vi "IMAQ-MWT Contour SPINE TEST (FPGA).vi"() -> ()   [LabVIEW 2015]
uses:
  <vilib>/Platform/TimedLoop/XDataNode/wakeup.ctl
  <vilib>/Platform/TimedLoop/XDataNode/XDNodeRunTimeDep.lvlib
  <vilib>/Platform/TimedLoop/XDataNode/nitl_modes.ctl
  <vilib>/Platform/TimedLoop/XDataNode/timing_clust.ctl
  <vilib>/Platform/TimedLoop/XDataNode/XDataNode.xnode
  <vilib>/rvi/DataTransferAndStorage/Container/XNode/niFpgaContainer.xnode
  <vilib>/rvi/interface/RandomDataEmulation/nirviRandomDataFpgaReadWriteTemplate.vi
panel:
  in  "Clock Cycles Limit":u32=10000
  # "IMAQ - MWT"
  # "Edge, Contour and SPINE"
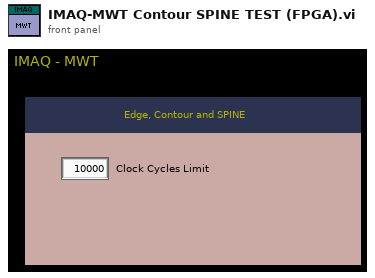
[diagram p1: front panel]
types:
  T1 = typedef "XDNodeRunTimeDep.lvlib/timing_clust.ctl" = cluster{"Expected End [f-1]":u64, "Actual End [f-1]":u64, "Finished Late? [f-1]":bool, "Expected End [i-1]":u64, "Actual End [i-1]":u64, "Finished Late? [i-1]":bool, "Expected Start [i]":u64, "Actual Start [i]":u64, "Expected Start [f]":u64, "Actual Start [f]":u64, "Source Name":string, "Structure Name":string, "Period":i64, "Deadline":i64, "Offset":i64, "Start":i64, "Priority":i32, "Timeout":i32, "Mode":T2, "Wakeup Reason":T3, "Error":errorcluster, "Source Type":string, "Secondary Source Type":string, "Global End Time":u64, "Global Start Time":u64, "Frame Duration":u64, "Iteration Duration":u64, "Assigned CPU":i32, "I/O Scan Engine Mode":u32}
  T2 = typedef "XDNodeRunTimeDep.lvlib/nitl_modes.ctl" = enum32{"No Change", "Process missed periods, maintain original phase", "Discard missed periods, maintain original phase", "Process missed periods, ignore original phase", "Discard missed periods, ignore original phase"}
  T3 = typedef "XDNodeRunTimeDep.lvlib/wakeup.ctl" = enum32{"Normal", "Aborted", "Asynchronous wakeup", "Timing source error", "Timed loop error", "Timeout"}
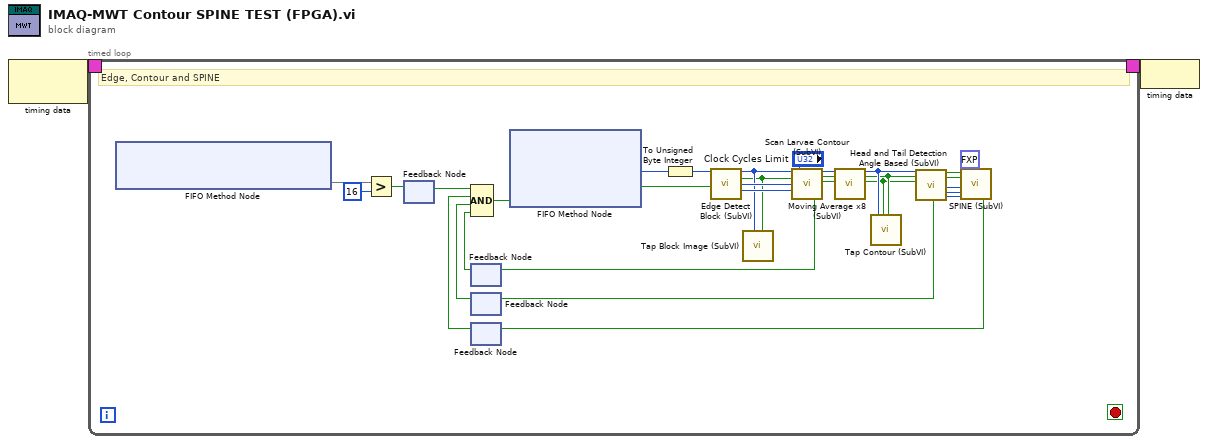
[diagram p0: block diagram]
diagram:
  n1 = node-c288() -> (w2:T1)  [unwired: 1 in]
  n2 = timed-loop {
    timing: w2 -> [_]
    timing-out: [_] -> w1
    stop <- _ stop-if-true
    # "Edge, Contour and SPINE"
    n3 = xnode ("FIFO Method Node")() -> ("Number of Elements to Write"=w17)  [unwired: 1 in, 1 out]
    n4 = Greater?(x=w17, y=u32 16) -> (0:w18:bool)
    n5 = feedback-in #1(w18) -> ()
    n6 = feedback #1() -> (w15:bool)  [unwired: 1 in]
    n7 = feedback #2() -> (w28:bool)  [unwired: 1 in]
    n8 = feedback #3() -> (w29:bool)  [unwired: 1 in]
    n9 = feedback #4() -> (w27:bool)  [unwired: 1 in]
    n10 = Compound Arithmetic op=AND(w15, w27, w29, w28) -> (w26:bool)
    n11 = xnode ("FIFO Method Node")("Ready for Output"=w26) -> ("Element"=w25:u64, "Output Valid"=w5:bool)  [unwired: 1 in, 1 out]
    n12 = To Unsigned Byte Integer(number=w25) -> (unsigned 8bit integer=w6:u8)
    n13 = call "Edge Detect Block (SubVI).vi"("Data In"=w6, "In Valid?"=w5) -> ("Data Out"=w4:u8, "Out Valid?"=w3:bool, "X Start"=w32:u16, "Y Start"=w33:u16)  [unwired: 10 in]
    n14 = call "Tap Block Image (SubVI).vi"("In Valid?"=w3, "Data In"=w4) -> ()  [unwired: 9 in, 1 out]
    n15 = call "Scan Larvae Contour (SubVI).vi"("Data In"=w4, "Input Valid?"=w3, "X Start"=w32, "Y Start"=w33, "Max. Scan Cycles"="Clock Cycles Limit") -> ("Ready for Input?"=w30:bool, "Boundary Point XY"=w24:u32, "Boundary Valid?"=w23:bool, "Scan End?"=w22:bool)  [unwired: 10 in, 1 out]
    n16 = feedback-in #2(w30) -> ()
    n17 = call "Moving Average x8 (SubVI).vi"("Point In"=w24, "Boundary Valid? In"=w23, "Scan End? In"=w22) -> ("Point Out"=w21:u32, "Boundary Valid? out"=w20:bool, "Scan End? Out"=w19:bool)  [unwired: 14 in]
    n18 = call "Tap Contour (SubVI).vi"("Contour XY"=w21, "Complete?"=w19, "Input Valid?"=w20) -> ()  [unwired: 17 in]
    n19 = call "Head and Tail Detection Angle Based (SubVI).vi"("Boundary Point XY"=w21, "Bondary Valid?"=w20, "Scan End?"=w19) -> ("Ready for Input?"=w8:bool, "Output Valid?"=w10:bool, "Skip Contour Analysis"=w11:bool, "V1 (ID)"=w12:u16, "V2 (ID)"=w13:u16, "N Points"=w14:u16)  [unwired: 9 in, 2 out]
    n20 = feedback-in #3(w8) -> ()
    n21 = call "SPINE (SubVI).vi"("Input Valid?"=w10, "Skip SPLINE?"=w11, "V1 (ID)"=w12, "V2 (ID)"=w13, "N Points"=w14, "N Spline Points"=fxp<+,8,8> 31.0) -> ("Ready for Input?"=w7:bool)  [unwired: 13 in]
    n22 = feedback-in #4(w7) -> ()
  }
  n23 = node-c288(w1) -> ()
